vi "ClusterToArray.vi"(8 "error in (no error)":errorcluster, 11 "RingdownConfig":T1={"Config"={"Addmod"=-1, "Scalmod"=0, "Lpocon"=-1, "Pircon"=-1, "Dmodes"=0, "Lpmcon"=3, "Lpacon"=1, "Fbcon"=1, "Ordcon"=1, "Trimre"=-1.0, "Ftrimh"=-1.0, "Ftriml"=-1.0}, "Window"={"StOffset"=1, "EndOffset"=601, "Length"=10000}, "V index"=0, "I index"=1, "PosSeq"=FALSE} {"Config"."Fbcon" items=["", "Forward", "Forward-Backward", "Backward"]; "Config"."Lpmcon" items=["", "Correlation", "Pre-windowed", "Covariance", "Post-windowed"]; "Config"."Lpacon" items=["", "SVD with possible rank reduction", "QR reduction via LAPACK", "Total least squares via SVD"]}) -> (0 "error out":errorcluster, 3 "RingdownInput":dbl[](array[numeric]))   [LabVIEW 2014, in "AppPlugins.lvlib" / "RingdownPlugin.lvclass"]
uses:
  RingdownPlugin.lvclass
  TypeDef/RingdownConfig.ctl
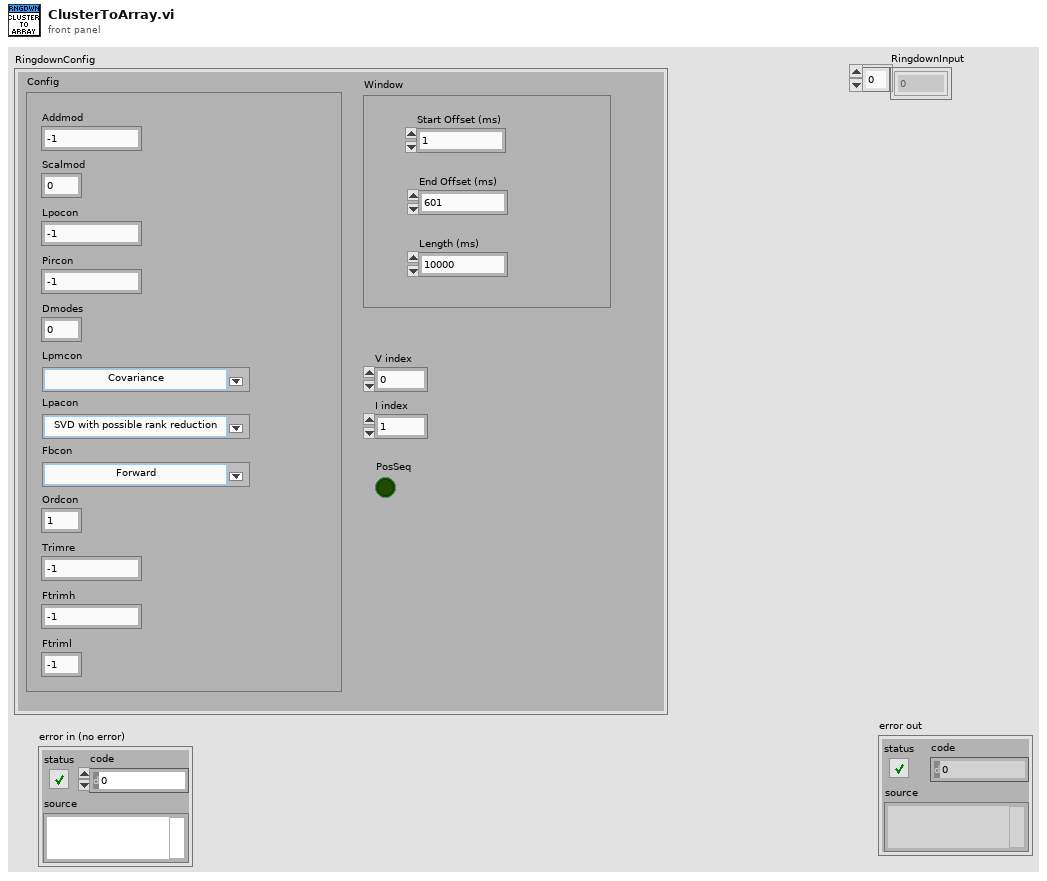
[diagram p1: front panel]
types:
  T1 = typedef "AppPlugins.lvlib/RingdownPlugin.lvclass/RingdownConfig.ctl" = cluster{"Config":cluster{"Addmod":i32, "Scalmod":i32, "Lpocon":i32, "Pircon":i32, "Dmodes":i32, "Lpmcon":u16, "Lpacon":u16, "Fbcon":u16, "Ordcon":i32, "Trimre":dbl, "Ftrimh":dbl, "Ftriml":dbl}, "Window":cluster{"StOffset":i32, "EndOffset":i32, "Length":i32}, "V index":i32, "I index":i32, "PosSeq":bool}
  T2 = cluster{"Addmod":i32, "Scalmod":i32, "Lpocon":i32, "Pircon":i32, "Dmodes":i32, "Lpmcon":u16, "Lpacon":u16, "Fbcon":u16, "Ordcon":i32, "Trimre":dbl, "Ftrimh":dbl, "Ftriml":dbl}
  T3 = cluster{"StOffset":i32, "EndOffset":i32, "Length":i32}
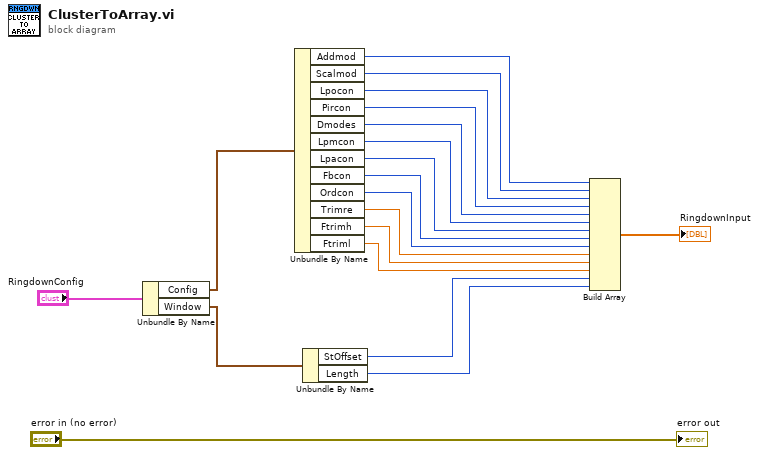
[diagram p0: block diagram]
diagram:
  n1 = Unbundle By Name("RingdownConfig") -> ("Config"=w18:T2, "Window"=w17:T3)
  n2 = Unbundle By Name(w18) -> ("Addmod"=w16:i32, "Scalmod"=w15:i32, "Lpocon"=w14:i32, "Pircon"=w13:i32, "Dmodes"=w12:i32, "Lpmcon"=w11:u16, "Lpacon"=w10:u16, "Fbcon"=w9:u16, "Ordcon"=w8:i32, "Trimre"=w7:dbl, "Ftrimh"=w6:dbl, "Ftriml"=w5:dbl)
  n3 = Unbundle By Name(w17) -> ("StOffset"=w4:i32, "Length"=w3:i32)
  n4 = Build Array(w16, w15, w14, w13, w12, w11, w10, w9, w8, w7, w6, w5, w4, w3) -> (→"RingdownInput":dbl[])
  "error out" <- "error in (no error)"
